vi "test TCX read (installed 71).vi"() -> ()   [LabVIEW 2011] (continued)
=\"http://www.garmin.com/xmlschemas/ActivityExtension/v2\"><Watts>106</Watts></TPX></Extensions></Trackpoint><Trackpoint><Time>2008-03-03T13:54:39Z</Time><Position><LatitudeDegrees>35.874921</LatitudeDegrees><LongitudeDegrees>-78.935340</LongitudeDegrees></Position><AltitudeMeters>93.385</AltitudeMeters><DistanceMeters>3447.353</DistanceMeters><Cadence>78</Cadence><Extensions><TPX xmlns=\"http://www.garmin.com/xmlschemas/ActivityExtension/v2\"><Watts>106</Watts></TPX></Extensions></Trackpoint><Trackpoint><Time>2008-03-03T13:54:40Z</Time><Position><LatitudeDegrees>35.874939</LatitudeDegrees><LongitudeDegrees>-78.935257</LongitudeDegrees></Position><AltitudeMeters>92.905</AltitudeMeters><DistanceMeters>3455.075</DistanceMeters><Cadence>78</Cadence><Extensions><TPX xmlns=\"http://www.garmin.com/xmlschemas/ActivityExtension/v2\"><Watts>107</Watts></TPX></Extensions></Trackpoint><Trackpoint><Time>2008-03-03T13:54:41Z</Time><Position><LatitudeDegrees>35.874959</LatitudeDegrees><LongitudeDegrees>-78.935174</LongitudeDegrees></Position><AltitudeMeters>92.905</AltitudeMeters><DistanceMeters>3462.864</DistanceMeters><Cadence>78</Cadence><Extensions><TPX xmlns=\"http://www.garmin.com/xmlschemas/ActivityExtension/v2\"><Watts>107</Watts></TPX></Extensions></Trackpoint><Trackpoint><Time>2008-03-03T13:54:42Z</Time><Position><LatitudeDegrees>35.874979</LatitudeDegrees><LongitudeDegrees>-78.935091</LongitudeDegrees></Position><AltitudeMeters>92.905</AltitudeMeters><DistanceMeters>3470.684</DistanceMeters><Cadence>79</Cadence><Extensions><TPX xmlns=\"http://www.garmin.com/xmlschemas/ActivityExtension/v2\"><Watts>102</Watts></TPX></Extensions></Trackpoint><Trackpoint><Time>2008-03-03T13:54:43Z</Time><Position><LatitudeDegrees>35.874999</LatitudeDegrees><LongitudeDegrees>-78.935010</LongitudeDegrees></Position><AltitudeMeters>92.905</AltitudeMeters><DistanceMeters>3478.419</DistanceMeters><Cadence>79</Cadence><Extensions><TPX xmlns=\"http://www.garmin.com/xmlschemas/ActivityExtension/v2\"><Watts>108</Watts></TPX></Extensions></Trackpoint><Trackpoint><Time>2008-03-03T13:54:44Z</Time><Position><LatitudeDegrees>35.875018</LatitudeDegrees><LongitudeDegrees>-78.934925</LongitudeDegrees></Position><AltitudeMeters>92.905</AltitudeMeters><DistanceMeters>3486.287</DistanceMeters><Cadence>75</Cadence><Extensions><TPX xmlns=\"http://www.garmin.com/xmlschemas/ActivityExtension/v2\"><Watts>106</Watts></TPX></Extensions></Trackpoint><Trackpoint><Time>2008-03-03T13:54:45Z</Time><Position><LatitudeDegrees>35.875035</LatitudeDegrees><LongitudeDegrees>-78.934840</LongitudeDegrees></Position><AltitudeMeters>92.424</AltitudeMeters><DistanceMeters>3494.270</DistanceMeters><Cadence>73</Cadence><Extensions><TPX xmlns=\"http://www.garmin.com/xmlschemas/ActivityExtension/v2\"><Watts>107</Watts></TPX></Extensions></Trackpoint><Trackpoint><Time>2008-03-03T13:54:46Z</Time><Position><LatitudeDegrees>35.875052</LatitudeDegrees><LongitudeDegrees>-78.934753</LongitudeDegrees></Position><AltitudeMeters>92.424</AltitudeMeters><DistanceMeters>3502.316</DistanceMeters><Cadence>73</Cadence><Extensions><TPX xmlns=\"http://www.garmin.com/xmlschemas/ActivityExtension/v2\"><Watts>109</Watts></TPX></Extensions></Trackpoint><Trackpoint><Time>2008-03-03T13:54:47Z</Time><Position><LatitudeDegrees>35.875069</LatitudeDegrees><LongitudeDegrees>-78.934665</LongitudeDegrees></Position><AltitudeMeters>92.424</AltitudeMeters><DistanceMeters>3510.458</DistanceMeters><Cadence>75</Cadence><Extensions><TPX xmlns=\"http://www.garmin.com/xmlschemas/ActivityExtension/v2\"><Watts>110</Watts></TPX></Extensions></Trackpoint><Trackpoint><Time>2008-03-03T13:54:48Z</Time><Position><LatitudeDegrees>35.875087</LatitudeDegrees><LongitudeDegrees>-78.934578</LongitudeDegrees></Position><AltitudeMeters>92.424</AltitudeMeters><DistanceMeters>3518.670</DistanceMeters><Cadence>76</Cadence><Extensions><TPX xmlns=\"http://www.garmin.com/xmlschemas/ActivityExtension/v2\"><Watts>111</Watts></TPX></Extensions></Trackpoint><Trackpoint><Time>2008-03-03T13:54:49Z</Time><Position><LatitudeDegrees>35.875104</LatitudeDegrees><LongitudeDegrees>-78.934486</LongitudeDegrees></Position><AltitudeMeters>92.424</AltitudeMeters><DistanceMeters>3527.182</DistanceMeters><Cadence>77</Cadence><Extensions><TPX xmlns=\"http://www.garmin.com/xmlschemas/ActivityExtension/v2\"><Watts>111</Watts></TPX></Extensions></Trackpoint><Trackpoint><Time>2008-03-03T13:54:50Z</Time><Position><LatitudeDegrees>35.875121</LatitudeDegrees><LongitudeDegrees>-78.934392</LongitudeDegrees></Position><AltitudeMeters>92.424</AltitudeMeters><DistanceMeters>3535.860</DistanceMeters><Cadence>79</Cadence><Extensions><TPX xmlns=\"http://www.garmin.com/xmlschemas/ActivityExtension/v2\"><Watts>111</Watts></TPX></Extensions></Trackpoint><Trackpoint><Time>2008-03-03T13:54:51Z</Time><Position><LatitudeDegrees>35.875137</LatitudeDegrees><LongitudeDegrees>-78.934295</LongitudeDegrees></Position><AltitudeMeters>91.943</AltitudeMeters><DistanceMeters>3544.788</DistanceMeters><Cadence>78</Cadence><Extensions><TPX xmlns=\"http://www.garmin.com/xmlschemas/ActivityExtension/v2\"><Watts>108</Watts></TPX></Extensions></Trackpoint><Trackpoint><Time>2008-03-03T13:54:52Z</Time><Position><LatitudeDegrees>35.875154</LatitudeDegrees><LongitudeDegrees>-78.934196</LongitudeDegrees></Position><AltitudeMeters>91.463</AltitudeMeters><DistanceMeters>3553.912</DistanceMeters><Cadence>74</Cadence><Extensions><TPX xmlns=\"http://www.garmin.com/xmlschemas/ActivityExtension/v2\"><Watts>103</Watts></TPX></Extensions></Trackpoint><Trackpoint><Time>2008-03-03T13:54:53Z</Time><Position><LatitudeDegrees>35.875172</LatitudeDegrees><LongitudeDegrees>-78.934096</LongitudeDegrees></Position><AltitudeMeters>91.463</AltitudeMeters><DistanceMeters>3563.297</DistanceMeters><Cadence>74</Cadence><Extensions><TPX xmlns=\"http://www.garmin.com/xmlschemas/ActivityExtension/v2\"><Watts>104</Watts></TPX></Extensions></Trackpoint><Trackpoint><Time>2008-03-03T13:54:54Z</Time><Position><LatitudeDegrees>35.875191</LatitudeDegrees><LongitudeDegrees>-78.933992</LongitudeDegrees></Position><AltitudeMeters>91.463</AltitudeMeters><DistanceMeters>3572.866</DistanceMeters><Cadence>77</Cadence><Extensions><TPX xmlns=\"http://www.garmin.com/xmlschemas/ActivityExtension/v2\"><Watts>118</Watts></TPX></Extensions></Trackpoint><Trackpoint><Time>2008-03-03T13:54:55Z</Time><Position><LatitudeDegrees>35.875211</LatitudeDegrees><LongitudeDegrees>-78.933885</LongitudeDegrees></Position><AltitudeMeters>90.982</AltitudeMeters><DistanceMeters>3582.741</DistanceMeters><Cadence>77</Cadence><Extensions><TPX xmlns=\"http://www.garmin.com/xmlschemas/ActivityExtension/v2\"><Watts>116</Watts></TPX></Extensions></Trackpoint><Trackpoint><Time>2008-03-03T13:54:56Z</Time><Position><LatitudeDegrees>35.875231</LatitudeDegrees><LongitudeDegrees>-78.933776</LongitudeDegrees></Position><AltitudeMeters>90.501</AltitudeMeters><DistanceMeters>3592.905</DistanceMeters><Cadence>73</Cadence><Extensions><TPX xmlns=\"http://www.garmin.com/xmlschemas/ActivityExtension/v2\"><Watts>109</Watts></TPX></Extensions></Trackpoint><Trackpoint><Time>2008-03-03T13:54:57Z</Time><Position><LatitudeDegrees>35.875253</LatitudeDegrees><LongitudeDegrees>-78.933665</LongitudeDegrees></Position><AltitudeMeters>90.501</AltitudeMeters><DistanceMeters>3603.271</DistanceMeters><Cadence>74</Cadence><Extensions><TPX xmlns=\"http://www.garmin.com/xmlschemas/ActivityExtension/v2\"><Watts>116</Watts></TPX></Extensions></Trackpoint><Trackpoint><Time>2008-03-03T13:54:58Z</Time><Position><LatitudeDegrees>35.875274</LatitudeDegrees><LongitudeDegrees>-78.933548</LongitudeDegrees></Position><AltitudeMeters>89.540</AltitudeMeters><DistanceMeters>3614.042</DistanceMeters><Cadence>74</Cadence><Extensions><TPX xmlns=\"http://www.garmin.com/xmlschemas/ActivityExtension/v2\"><Watts>115</Watts></TPX></Extensions></Trackpoint><Trackpoint><Time>2008-03-03T13:54:59Z</Time><Position><LatitudeDegrees>35.875302</LatitudeDegrees><LongitudeDegrees>-78.933428</LongitudeDegrees></Position><AltitudeMeters>88.579</AltitudeMeters><DistanceMeters>3625.394</DistanceMeters><Cadence>77</Cadence><Extensions><TPX xmlns=\"http://www.garmin.com/xmlschemas/ActivityExtension/v2\"><Watts>111</Watts></TPX></Extensions></Trackpoint><Trackpoint><Time>2008-03-03T13:55:00Z</Time><Position><LatitudeDegrees>35.875328</LatitudeDegrees><LongitudeDegrees>-78.933302</LongitudeDegrees></Position><AltitudeMeters>87.617</AltitudeMeters><DistanceMeters>3637.135</DistanceMeters><Cadence>83</Cadence><Extensions><TPX xmlns=\"http://www.garmin.com/xmlschemas/ActivityExtension/v2\"><Watts>111</Watts></TPX></Extensions></Trackpoint><Trackpoint><Time>2008-03-03T13:55:01Z</Time><Position><LatitudeDegrees>35.875352</LatitudeDegrees><LongitudeDegrees>-78.933170</LongitudeDegrees></Position><AltitudeMeters>86.656</AltitudeMeters><DistanceMeters>3649.341</DistanceMeters><Cadence>87</Cadence><Extensions><TPX xmlns=\"http://www.garmin.com/xmlschemas/ActivityExtension/v2\"><Watts>108</Watts></TPX></Extensions></Trackpoint><Trackpoint><Time>2008-03-03T13:55:02Z</Time><Position><LatitudeDegrees>35.875375</LatitudeDegrees><LongitudeDegrees>-78.933034</LongitudeDegrees></Position><AltitudeMeters>86.175</AltitudeMeters><DistanceMeters>3661.935</DistanceMeters><Cadence>77</Cadence><Extensions><TPX xmlns=\"http://www.garmin.com/xmlschemas/ActivityExtension/v2\"><Watts>105</Watts></TPX></Extensions></Trackpoint><Trackpoint><Time>2008-03-03T13:55:03Z</Time><Position><LatitudeDegrees>35.875397</LatitudeDegrees><LongitudeDegrees>-78.932892</LongitudeDegrees></Position><AltitudeMeters>85.695</AltitudeMeters><DistanceMeters>3675.075</DistanceMeters><Cadence>77</Cadence><Extensions><TPX xmlns=\"http://www.garmin.com/xmlschemas/ActivityExtension/v2\"><Watts>106</Watts></TPX></Extensions></Trackpoint><Trackpoint><Time>2008-03-03T13:55:04Z</Time><Position><LatitudeDegrees>35.875423</LatitudeDegrees><LongitudeDegrees>-78.932744</LongitudeDegrees></Position><AltitudeMeters>84.733</AltitudeMeters><DistanceMeters>3688.721</DistanceMeters><Cadence>81</Cadence><Extensions><TPX xmlns=\"http://www.garmin.com/xmlschemas/ActivityExtension/v2\"><Watts>109</Watts></TPX></Extensions></Trackpoint><Trackpoint><Time>2008-03-03T13:55:05Z</Time><Position><LatitudeDegrees>35.875451</LatitudeDegrees><LongitudeDegrees>-78.932591</LongitudeDegrees></Position><AltitudeMeters>83.772</AltitudeMeters><DistanceMeters>3702.913</DistanceMeters><Cadence>84</Cadence><Extensions><TPX xmlns=\"http://www.garmin.com/xmlschemas/ActivityExtension/v2\"><Watts>130</Watts></TPX></Extensions></Trackpoint><Trackpoint><Time>2008-03-03T13:55:06Z</Time><Position><LatitudeDegrees>35.875484</LatitudeDegrees><LongitudeDegrees>-78.932435</LongitudeDegrees></Position><AltitudeMeters>83.291</AltitudeMeters><DistanceMeters>3717.524</DistanceMeters><Cadence>87</Cadence><Extensions><TPX xmlns=\"http://www.garmin.com/xmlschemas/ActivityExtension/v2\"><Watts>156</Watts></TPX></Extensions></Trackpoint><Trackpoint><Time>2008-03-03T13:55:07Z</Time><Position><LatitudeDegrees>35.875516</LatitudeDegrees><LongitudeDegrees>-78.932275</LongitudeDegrees></Position><AltitudeMeters>82.811</AltitudeMeters><DistanceMeters>3732.393</DistanceMeters><Cadence>89</Cadence><Extensions><TPX xmlns=\"http://www.garmin.com/xmlschemas/ActivityExtension/v2\"><Watts>168</Watts></TPX></Extensions></Trackpoint><Trackpoint><Time>2008-03-03T13:55:08Z</Time><Position><LatitudeDegrees>35.875546</LatitudeDegrees><LongitudeDegrees>-78.932113</LongitudeDegrees></Position><AltitudeMeters>81.849</AltitudeMeters><DistanceMeters>3747.414</DistanceMeters><Cadence>90</Cadence><Extensions><TPX xmlns=\"http://www.garmin.com/xmlschemas/ActivityExtension/v2\"><Watts>157</Watts></TPX></Extensions></Trackpoint><Trackpoint><Time>2008-03-03T13:55:09Z</Time><Position><LatitudeDegrees>35.875574</LatitudeDegrees><LongitudeDegrees>-78.931949</LongitudeDegrees></Position><AltitudeMeters>80.888</AltitudeMeters><DistanceMeters>3762.486</DistanceMeters><Cadence>89</Cadence><Extensions><TPX xmlns=\"http://www.garmin.com/xmlschemas/ActivityExtension/v2\"><Watts>146</Watts></TPX></Extensions></Trackpoint><Trackpoint><Time>2008-03-03T13:55:10Z</Time><Position><LatitudeDegrees>35.875600</LatitudeDegrees><LongitudeDegrees>-78.931785</LongitudeDegrees></Position><AltitudeMeters>80.407</AltitudeMeters><DistanceMeters>3777.574</DistanceMeters><Cadence>89</Cadence><Extensions><TPX xmlns=\"http://www.garmin.com/xmlschemas/ActivityExtension/v2\"><Watts>134</Watts></TPX></Extensions></Trackpoint><Trackpoint><Time>2008-03-03T13:55:11Z</Time><Position><LatitudeDegrees>35.875627</LatitudeDegrees><LongitudeDegrees>-78.931623</LongitudeDegrees></Position><AltitudeMeters>79.446</AltitudeMeters><DistanceMeters>3792.520</DistanceMeters><Cadence>89</Cadence><Extensions><TPX xmlns=\"http://www.garmin.com/xmlschemas/ActivityExtension/v2\"><Watts>130</Watts></TPX></Extensions></Trackpoint><Trackpoint><Time>2008-03-03T13:55:12Z</Time><Position><LatitudeDegrees>35.875652</LatitudeDegrees><LongitudeDegrees>-78.931459</LongitudeDegrees></Position><AltitudeMeters>79.446</AltitudeMeters><DistanceMeters>3807.590</DistanceMeters><Cadence>88</Cadence><Extensions><TPX xmlns=\"http://www.garmin.com/xmlschemas/ActivityExtension/v2\"><Watts>124</Watts></TPX></Extensions></Trackpoint><Trackpoint><Time>2008-03-03T13:55:13Z</Time><Position><LatitudeDegrees>35.875671</LatitudeDegrees><LongitudeDegrees>-78.931297</LongitudeDegrees></Position><AltitudeMeters>78.965</AltitudeMeters><DistanceMeters>3822.386</DistanceMeters><Cadence>88</Cadence><Extensions><TPX xmlns=\"http://www.garmin.com/xmlschemas/ActivityExtension/v2\"><Watts>124</Watts></TPX></Extensions></Trackpoint><Trackpoint><Time>2008-03-03T13:55:14Z</Time><Position><LatitudeDegrees>35.875682</LatitudeDegrees><LongitudeDegrees>-78.931138</LongitudeDegrees></Position><AltitudeMeters>78.004</AltitudeMeters><DistanceMeters>3836.777</DistanceMeters><Cadence>86</Cadence><Extensions><TPX xmlns=\"http://www.garmin.com/xmlschemas/ActivityExtension/v2\"><Watts>122</Watts></TPX></Extensions></Trackpoint><Trackpoint><Time>2008-03-03T13:55:15Z</Time><Position><LatitudeDegrees>35.875686</LatitudeDegrees><LongitudeDegrees>-78.930981</LongitudeDegrees></Position><AltitudeMeters>78.004</AltitudeMeters><DistanceMeters>3850.902</DistanceMeters><Cadence>85</Cadence><Extensions><TPX xmlns=\"http://www.garmin.com/xmlschemas/ActivityExtension/v2\"><Watts>136</Watts></TPX></Extensions></Trackpoint><Trackpoint><Time>2008-03-03T13:55:16Z</Time><Position><LatitudeDegrees>35.875685</LatitudeDegrees><LongitudeDegrees>-78.930828</LongitudeDegrees></Position><AltitudeMeters>78.004</AltitudeMeters><DistanceMeters>3864.689</DistanceMeters><Cadence>83</Cadence><Extensions><TPX xmlns=\"http://www.garmin.com/xmlschemas/ActivityExtension/v2\"><Watts>148</Watts></TPX></Extensions></Trackpoint><Trackpoint><Time>2008-03-03T13:55:17Z</Time><Position><LatitudeDegrees>35.875684</LatitudeDegrees><LongitudeDegrees>-78.930679</LongitudeDegrees></Position><AltitudeMeters>77.523</AltitudeMeters><DistanceMeters>3878.168</DistanceMeters><Cadence>80</Cadence><Extensions><TPX xmlns=\"http://www.garmin.com/xmlschemas/ActivityExtension/v2\"><Watts>165</Watts></TPX></Extensions></Trackpoint><Trackpoint><Time>2008-03-03T13:55:18Z</Time><Position><LatitudeDegrees>35.875681</LatitudeDegrees><LongitudeDegrees>-78.930532</LongitudeDegrees></Position><AltitudeMeters>77.043</AltitudeMeters><DistanceMeters>3891.426</DistanceMeters><Cadence>79</Cadence><Extensions><TPX xmlns=\"http://www.garmin.com/xmlschemas/ActivityExtension/v2\"><Watts>164</Watts></TPX></Extensions></Trackpoint><Trackpoint><Time>2008-03-03T13:55:19Z</Time><Position><LatitudeDegrees>35.875675</LatitudeDegrees><LongitudeDegrees>-78.930389</LongitudeDegrees></Position><AltitudeMeters>77.043</AltitudeMeters><DistanceMeters>3904.342</DistanceMeters><Cadence>78</Cadence><Extensions><TPX xmlns=\"http://www.garmin.com/xmlschemas/ActivityExtension/v2\"><Watts>161</Watts></TPX></Extensions></Trackpoint><Trackpoint><Time>2008-03-03T13:55:20Z</Time><Position><LatitudeDegrees>35.875671</LatitudeDegrees><LongitudeDegrees>-78.930247</LongitudeDegrees></Position><AltitudeMeters>76.562</AltitudeMeters><DistanceMeters>3917.112</DistanceMeters><Cadence>76</Cadence><Extensions><TPX xmlns=\"http://www.garmin.com/xmlschemas/ActivityExtension/v2\"><Watts>154</Watts></TPX></Extensions></Trackpoint><Trackpoint><Time>2008-03-03T13:55:21Z</Time><Position><LatitudeDegrees>35.875667</LatitudeDegrees><LongitudeDegrees>-78.930109</LongitudeDegrees></Position><AltitudeMeters>78.004</AltitudeMeters><DistanceMeters>3929.621</DistanceMeters><Cadence>75</Cadence><Extensions><TPX xmlns=\"http://www.garmin.com/xmlschemas/ActivityExtension/v2\"><Watts>160</Watts></TPX></Extensions></Trackpoint><Trackpoint><Time>2008-03-03T13:55:22Z</Time><Position><LatitudeDegrees>35.875662</LatitudeDegrees><LongitudeDegrees>-78.929972</LongitudeDegrees></Position><AltitudeMeters>77.043</AltitudeMeters><DistanceMeters>3941.995</DistanceMeters><Cadence>74</Cadence><Extensions><TPX xmlns=\"http://www.garmin.com/xmlschemas/ActivityExtension/v2\"><Watts>164</Watts></TPX></Extensions></Trackpoint><Trackpoint><Time>2008-03-03T13:55:23Z</Time><Position><LatitudeDegrees>35.875657</LatitudeDegrees><LongitudeDegrees>-78.929836</LongitudeDegrees></Position><AltitudeMeters>76.562</AltitudeMeters><DistanceMeters>3954.253</DistanceMeters><Cadence>74</Cadence><Extensions><TPX xmlns=\"http://www.garmin.com/xmlschemas/ActivityExtension/v2\"><Watts>162</Watts></TPX></Extensions></Trackpoint><Trackpoint><Time>2008-03-03T13:55:24Z</Time><Position><LatitudeDegrees>35.875652</LatitudeDegrees><LongitudeDegrees>-78.929703</LongitudeDegrees></Position><AltitudeMeters>76.562</AltitudeMeters><DistanceMeters>3966.223</DistanceMeters><Cadence>72</Cadence><Extensions><TPX xmlns=\"http://www.garmin.com/xmlschemas/ActivityExtension/v2\"><Watts>178</Watts></TPX></Extensions></Trackpoint><Trackpoint><Time>2008-03-03T13:55:25Z</Time><Position><LatitudeDegrees>35.875651</LatitudeDegrees><LongitudeDegrees>-78.929573</LongitudeDegrees></Position><AltitudeMeters>76.081</AltitudeMeters><DistanceMeters>3978.047</DistanceMeters><Cadence>72</Cadence><Extensions><TPX xmlns=\"http://www.garmin.com/xmlschemas/ActivityExtension/v2\"><Watts>180</Watts></TPX></Extensions></Trackpoint><Trackpoint><Time>2008-03-03T13:55:26Z</Time><Position><LatitudeDegrees>35.875647</LatitudeDegrees><LongitudeDegrees>-78.929443</LongitudeDegrees></Position><AltitudeMeters>76.081</AltitudeMeters><DistanceMeters>3989.714</DistanceMeters><Cadence>71</Cadence><Extensions><TPX xmlns=\"http://www.garmin.com/xmlschemas/ActivityExtension/v2\"><Watts>192</Watts></TPX></Extensions></Trackpoint><Trackpoint><Time>2008-03-03T13:55:27Z</Time><Position><LatitudeDegrees>35.875640</LatitudeDegrees><LongitudeDegrees>-78.929316</LongitudeDegrees></Position><AltitudeMeters>76.562</AltitudeMeters><DistanceMeters>4001.237</DistanceMeters><Cadence>69</Cadence><Extensions><TPX xmlns=\"http://www.garmin.com/xmlschemas/ActivityExtension/v2\"><Watts>191</Watts></TPX></Extensions></Trackpoint><Trackpoint><Time>2008-03-03T13:55:28Z</Time><Position><LatitudeDegrees>35.875631</LatitudeDegrees><LongitudeDegrees>-78.929192</LongitudeDegrees></Position><AltitudeMeters>77.043</AltitudeMeters><DistanceMeters>4012.524</DistanceMeters><Cadence>68</Cadence><Extensions><TPX xmlns=\"http://www.garmin.com/xmlschemas/ActivityExtension/v2\"><Watts>166</Watts></TPX></Extensions></Trackpoint><Trackpoint><Time>2008-03-03T13:55:29Z</Time><Position><LatitudeDegrees>35.875625</LatitudeDegrees><LongitudeDegrees>-78.929072</LongitudeDegrees></Position><AltitudeMeters>77.043</AltitudeMeters><DistanceMeters>4023.291</DistanceMeters><Cadence>66</Cadence><Extensions><TPX xmlns=\"http://www.garmin.com/xmlschemas/ActivityExtension/v2\"><Watts>142</Watts></TPX></Extensions></Trackpoint><Trackpoint><Time>2008-03-03T13:55:30Z</Time><Position><LatitudeDegrees>35.875618</LatitudeDegrees><LongitudeDegrees>-78.928955</LongitudeDegrees></Position><AltitudeMeters>76.562</AltitudeMeters><DistanceMeters>4033.810</DistanceMeters><Cadence>66</Cadence><Extensions><TPX xmlns=\"http://www.garmin.com/xmlschemas/ActivityExtension/v2\"><Watts>142</Watts></TPX></Extensions></Trackpoint><Trackpoint><Time>2008-03-03T13:55:31Z</Time><Position><LatitudeDegrees>35.875612</LatitudeDegrees><LongitudeDegrees>-78.928844</LongitudeDegrees></Position><AltitudeMeters>76.562</AltitudeMeters><DistanceMeters>4043.911</DistanceMeters><Cadence>68</Cadence><Extensions><TPX xmlns=\"http://www.garmin.com/xmlschemas/ActivityExtension/v2\"><Watts>145</Watts></TPX></Extensions></Trackpoint><Trackpoint><Time>2008-03-03T13:55:32Z</Time><Position><LatitudeDegrees>35.875608</LatitudeDegrees><LongitudeDegrees>-78.928738</LongitudeDegrees></Position><AltitudeMeters>77.043</AltitudeMeters><DistanceMeters>4053.442</DistanceMeters><Cadence>68</Cadence><Extensions><TPX xmlns=\"http://www.garmin.com/xmlschemas/ActivityExtension/v2\"><Watts>151</Watts></TPX></Extensions></Trackpoint><Trackpoint><Time>2008-03-03T13:55:33Z</Time><Position><LatitudeDegrees>35.875606</LatitudeDegrees><LongitudeDegrees>-78.928635</LongitudeDegrees></Position><AltitudeMeters>77.523</AltitudeMeters><DistanceMeters>4062.742</DistanceMeters><Cadence>68</Cadence><Extensions><TPX xmlns=\"http://www.garmin.com/xmlschemas/ActivityExtension/v2\"><Watts>149</Watts></TPX></Extensions></Trackpoint><Trackpoint><Time>2008-03-03T13:55:34Z</Time><Position><LatitudeDegrees>35.875603</LatitudeDegrees><LongitudeDegrees>-78.928536</LongitudeDegrees></Position><AltitudeMeters>78.004</AltitudeMeters><DistanceMeters>4071.697</DistanceMeters><Cadence>65</Cadence><Extensions><TPX xmlns=\"http://www.garmin.com/xmlschemas/ActivityExtension/v2\"><Watts>312</Watts></TPX></Extensions></Trackpoint><Trackpoint><Time>2008-03-03T13:55:35Z</Time><Position><LatitudeDegrees>35.875600</LatitudeDegrees><LongitudeDegrees>-78.928438</LongitudeDegrees></Position><AltitudeMeters>78.485</AltitudeMeters><DistanceMeters>4080.494</DistanceMeters><Cadence>65</Cadence><Extensions><TPX xmlns=\"http://www.garmin.com/xmlschemas/ActivityExtension/v2\"><Watts>316</Watts></TPX></Extensions></Trackpoint><Trackpoint><Time>2008-03-03T13:55:36Z</Time><Position><LatitudeDegrees>35.875592</LatitudeDegrees><LongitudeDegrees>-78.928342</LongitudeDegrees></Position><AltitudeMeters>78.485</AltitudeMeters><DistanceMeters>4089.234</DistanceMeters><Cadence>63</Cadence><Extensions><TPX xmlns=\"http://www.garmin.com/xmlschemas/ActivityExtension/v2\"><Watts>338</Watts></TPX></Extensions></Trackpoint><Trackpoint><Time>2008-03-03T13:55:37Z</Time><Position><LatitudeDegrees>35.875583</LatitudeDegrees><LongitudeDegrees>-78.928247</LongitudeDegrees></Position><AltitudeMeters>78.965</AltitudeMeters><DistanceMeters>4097.860</DistanceMeters><Cadence>62</Cadence><Extensions><TPX xmlns=\"http://www.garmin.com/xmlschemas/ActivityExtension/v2\"><Watts>355</Watts></TPX></Extensions></Trackpoint><Trackpoint><Time>2008-03-03T13:55:38Z</Time><Position><LatitudeDegrees>35.875580</LatitudeDegrees><LongitudeDegrees>-78.928153</LongitudeDegrees></Position><AltitudeMeters>79.446</AltitudeMeters><DistanceMeters>4106.294</DistanceMeters><Cadence>61</Cadence><Extensions><TPX xmlns=\"http://www.garmin.com/xmlschemas/ActivityExtension/v2\"><Watts>372</Watts></TPX></Extensions></Trackpoint><Trackpoint><Time>2008-03-03T13:55:39Z</Time><Position><LatitudeDegrees>35.875570</LatitudeDegrees><LongitudeDegrees>-78.928059</LongitudeDegrees></Position><AltitudeMeters>79.446</AltitudeMeters><DistanceMeters>4114.865</DistanceMeters><Cadence>61</Cadence><Extensions><TPX xmlns=\"http://www.garmin.com/xmlschemas/ActivityExtension/v2\"><Watts>376</Watts></TPX></Extensions></Trackpoint><Trackpoint><Time>2008-03-03T13:55:40Z</Time><Position><LatitudeDegrees>35.875562</LatitudeDegrees><LongitudeDegrees>-78.927965</LongitudeDegrees></Position><AltitudeMeters>79.927</AltitudeMeters><DistanceMeters>4123.438</DistanceMeters><Cadence>61</Cadence><Extensions><TPX xmlns=\"http://www.garmin.com/xmlschemas/ActivityExtension/v2\"><Watts>374</Watts></TPX></Extensions></Trackpoint><Trackpoint><Time>2008-03-03T13:55:41Z</Time><Position><LatitudeDegrees>35.875555</LatitudeDegrees><LongitudeDegrees>-78.927871</LongitudeDegrees></Position><AltitudeMeters>79.927</AltitudeMeters><DistanceMeters>4131.906</DistanceMeters><Cadence>61</Cadence><Extensions><TPX xmlns=\"http://www.garmin.com/xmlschemas/ActivityExtension/v2\"><Watts>375</Watts></TPX></Extensions></Trackpoint><Trackpoint><Time>2008-03-03T13:55:42Z</Time><Position><LatitudeDegrees>35.875548</LatitudeDegrees><LongitudeDegrees>-78.927776</LongitudeDegrees></Position><AltitudeMeters>79.927</AltitudeMeters><DistanceMeters>4140.581</DistanceMeters><Cadence>62</Cadence><Extensions><TPX xmlns=\"http://www.garmin.com/xmlschemas/ActivityExtension/v2\"><Watts>335</Watts></TPX></Extensions></Trackpoint><Trackpoint><Time>2008-03-03T13:55:43Z</Time><Position><LatitudeDegrees>35.875543</LatitudeDegrees><LongitudeDegrees>-78.927681</LongitudeDegrees></Position><AltitudeMeters>80.407</AltitudeMeters><DistanceMeters>4149.183</DistanceMeters><Cadence>62</Cadence><Extensions><TPX xmlns=\"http://www.garmin.com/xmlschemas/ActivityExtension/v2\"><Watts>289</Watts></TPX></Extensions></Trackpoint><Trackpoint><Time>2008-03-03T13:55:44Z</Time><Position><LatitudeDegrees>35.875535</LatitudeDegrees><LongitudeDegrees>-78.927586</LongitudeDegrees></Position><AltitudeMeters>80.407</AltitudeMeters><DistanceMeters>4157.797</DistanceMeters><Cadence>62</Cadence><Extensions><TPX xmlns=\"http://www.garmin.com/xmlschemas/ActivityExtension/v2\"><Watts>224</Watts></TPX></Extensions></Trackpoint><Trackpoint><Time>2008-03-03T13:55:45Z</Time><Position><LatitudeDegrees>35.875521</LatitudeDegrees><LongitudeDegrees>-78.927489</LongitudeDegrees></Position><AltitudeMeters>80.407</AltitudeMeters><DistanceMeters>4166.648</DistanceMeters><Cadence>62</Cadence><Extensions><TPX xmlns=\"http://www.garmin.com/xmlschemas/ActivityExtension/v2\"><Watts>223</Watts></TPX></Extensions></Trackpoint><Trackpoint><Time>2008-03-03T13:55:46Z</Time><Position><LatitudeDegrees>35.875508</LatitudeDegrees><LongitudeDegrees>-78.927391</LongitudeDegrees></Position><AltitudeMeters>79.927</AltitudeMeters><DistanceMeters>4175.647</DistanceMeters><Cadence>63</Cadence><Extensions><TPX xmlns=\"http://www.garmin.com/xmlschemas/ActivityExtension/v2\"><Watts>210</Watts></TPX></Extensions></Trackpoint><Trackpoint><Time>2008-03-03T13:55:47Z</Time><Position><LatitudeDegrees>35.875496</LatitudeDegrees><LongitudeDegrees>-78.927292</LongitudeDegrees></Position><AltitudeMeters>79.927</AltitudeMeters><DistanceMeters>4184.702</DistanceMeters><Cadence>63</Cadence><Extensions><TPX xmlns=\"http://www.garmin.com/xmlschemas/ActivityExtension/v2\"><Watts>206</Watts></TPX></Extensions></Trackpoint><Trackpoint><Time>2008-03-03T13:55:48Z</Time><Position><LatitudeDegrees>35.875484</LatitudeDegrees><LongitudeDegrees>-78.927191</LongitudeDegrees></Position><AltitudeMeters>79.927</AltitudeMeters><DistanceMeters>4193.944</DistanceMeters><Cadence>64</Cadence><Extensions><TPX xmlns=\"http://www.garmin.com/xmlschemas/ActivityExtension/v2\"><Watts>175</Watts></TPX></Extensions></Trackpoint><Trackpoint><Time>2008-03-03T13:55:49Z</Time><Position><LatitudeDegrees>35.875472</LatitudeDegrees><LongitudeDegrees>-78.927087</LongitudeDegrees></Position><AltitudeMeters>78.965</AltitudeMeters><DistanceMeters>4203.405</DistanceMeters><Cadence>67</Cadence><Extensions><TPX xmlns=\"http://www.garmin.com/xmlschemas/ActivityExtension/v2\"><Watts>118</Watts></TPX></Extensions></Trackpoint><Trackpoint><Time>2008-03-03T13:55:50Z</Time><Position><LatitudeDegrees>35.875459</LatitudeDegrees><LongitudeDegrees>-78.926981</LongitudeDegrees></Position><AltitudeMeters>79.446</AltitudeMeters><DistanceMeters>4213.108</DistanceMeters><Cadence>69</Cadence><Extensions><TPX xmlns=\"http://www.garmin.com/xmlschemas/ActivityExtension/v2\"><Watts>109</Watts></TPX></Extensions></Trackpoint><Trackpoint><Time>2008-03-03T13:55:51Z</Time><Position><LatitudeDegrees>35.875446</LatitudeDegrees><LongitudeDegrees>-78.926870</LongitudeDegrees></Position><AltitudeMeters>78.485</AltitudeMeters><DistanceMeters>4223.207</DistanceMeters><Cadence>71</Cadence><Extensions><TPX xmlns=\"http://www.garmin.com/xmlschemas/ActivityExtension/v2\"><Watts>106</Watts></TPX></Extensions></Trackpoint><Trackpoint><Time>2008-03-03T13:55:52Z</Time><Position><LatitudeDegrees>35.875433</LatitudeDegrees><LongitudeDegrees>-78.926755</LongitudeDegrees></Position><AltitudeMeters>78.485</AltitudeMeters><DistanceMeters>4233.738</DistanceMeters><Cadence>71</Cadence><Extensions><TPX xmlns=\"http://www.garmin.com/xmlschemas/ActivityExtension/v2\"><Watts>107</Watts></TPX></Extensions></Trackpoint><Trackpoint><Time>2008-03-03T13:55:53Z</Time><Position><LatitudeDegrees>35.875420</LatitudeDegrees><LongitudeDegrees>-78.926635</LongitudeDegrees></Position><AltitudeMeters>78.004</AltitudeMeters><DistanceMeters>4244.720</DistanceMeters><Cadence>79</Cadence><Extensions><TPX xmlns=\"http://www.garmin.com/xmlschemas/ActivityExtension/v2\"><Watts>106</Watts></TPX></Extensions></Trackpoint><Trackpoint><Time>2008-03-03T13:55:54Z</Time><Position><LatitudeDegrees>35.875406</LatitudeDegrees><LongitudeDegrees>-78.926511</LongitudeDegrees></Position><AltitudeMeters>77.043</AltitudeMeters><DistanceMeters>4256.063</DistanceMeters><Cadence>81</Cadence><Extensions><TPX xmlns=\"http://www.garmin.com/xmlschemas/ActivityExtension/v2\"><Watts>108</Watts></TPX></Extensions></Trackpoint><Trackpoint><Time>2008-03-03T13:55:55Z</Time><Position><LatitudeDegrees>35.875394</LatitudeDegrees><LongitudeDegrees>-78.926382</LongitudeDegrees></Position><AltitudeMeters>76.562</AltitudeMeters><DistanceMeters>4267.799</DistanceMeters><Cadence>84</Cadence><Extensions><TPX xmlns=\"http://www.garmin.com/xmlschemas/ActivityExtension/v2\"><Watts>102</Watts></TPX></Extensions></Trackpoint><Trackpoint><Time>2008-03-03T13:55:56Z</Time><Position><LatitudeDegrees>35.875387</LatitudeDegrees><LongitudeDegrees>-78.926251</LongitudeDegrees></Position><AltitudeMeters>76.562</AltitudeMeters><DistanceMeters>4279.712</DistanceMeters><Cadence>85</Cadence><Extensions><TPX xmlns=\"http://www.garmin.com/xmlschemas/ActivityExtension/v2\"><Watts>103</Watts></TPX></Extensions></Trackpoint><Trackpoint><Time>2008-03-03T13:55:57Z</Time><Position><LatitudeDegrees>35.875381</LatitudeDegrees><LongitudeDegrees>-78.926117</LongitudeDegrees></Position><AltitudeMeters>76.562</AltitudeMeters><DistanceMeters>4291.779</DistanceMeters><Cadence>85</Cadence><Extensions><TPX xmlns=\"http://www.garmin.com/xmlschemas/ActivityExtension/v2\"><Watts>102</Watts></TPX></Extensions></Trackpoint><Trackpoint><Time>2008-03-03T13:55:58Z</Time><Position><LatitudeDegrees>35.875374</LatitudeDegrees><LongitudeDegrees>-78.925982</LongitudeDegrees></Position><AltitudeMeters>76.081</AltitudeMeters><DistanceMeters>4304.011</DistanceMeters><Cadence>85</Cadence><Extensions><TPX xmlns=\"http://www.garmin.com/xmlschemas/ActivityExtension/v2\"><Watts>107</Watts></TPX></Extensions></Trackpoint><Trackpoint><Time>2008-03-03T13:55:59Z</Time><Position><LatitudeDegrees>35.875372</LatitudeDegrees><LongitudeDegrees>-78.925849</LongitudeDegrees></Position><AltitudeMeters>75.120</AltitudeMeters><DistanceMeters>4316.005</DistanceMeters><Cadence>84</Cadence><Extensions><TPX xmlns=\"http://www.garmin.com/xmlschemas/ActivityExtension/v2\"><Watts>105</Watts></TPX></Extensions></Trackpoint><Trackpoint><Time>2008-03-03T13:56:00Z</Time><Position><LatitudeDegrees>35.875374</LatitudeDegrees><LongitudeDegrees>-78.925719</LongitudeDegrees></Position><AltitudeMeters>74.640</AltitudeMeters><DistanceMeters>4327.800</DistanceMeters><Cadence>83</Cadence><Extensions><TPX xmlns=\"http://www.garmin.com/xmlschemas/ActivityExtension/v2\"><Watts>108</Watts></TPX></Extensions></Trackpoint><Trackpoint><Time>2008-03-03T13:56:01Z</Time><Position><LatitudeDegrees>35.875377</LatitudeDegrees><LongitudeDegrees>-78.925590</LongitudeDegrees></Position><AltitudeMeters>74.640</AltitudeMeters><DistanceMeters>4339.303</DistanceMeters><Cadence>81</Cadence><Extensions><TPX xmlns=\"http://www.garmin.com/xmlschemas/ActivityExtension/v2\"><Watts>111</Watts></TPX></Extensions></Trackpoint><Trackpoint><Time>2008-03-03T13:56:02Z</Time><Position><LatitudeDegrees>35.875376</LatitudeDegrees><LongitudeDegrees>-78.925464</LongitudeDegrees></Position><AltitudeMeters>74.159</AltitudeMeters><DistanceMeters>4350.667</DistanceMeters><Cadence>81</Cadence><Extensions><TPX xmlns=\"http://www.garmin.com/xmlschemas/ActivityExtension/v2\"><Watts>110</Watts></TPX></Extensions></Trackpoint><Trackpoint><Time>2008-03-03T13:56:03Z</Time><Position><LatitudeDegrees>35.875378</LatitudeDegrees><LongitudeDegrees>-78.925342</LongitudeDegrees></Position><AltitudeMeters>74.640</AltitudeMeters><DistanceMeters>4361.797</DistanceMeters><Cadence>79</Cadence><Extensions><TPX xmlns=\"http://www.garmin.com/xmlschemas/ActivityExtension/v2\"><Watts>111</Watts></TPX></Extensions></Trackpoint><Trackpoint><Time>2008-03-03T13:56:04Z</Time><Position><LatitudeDegrees>35.875384</LatitudeDegrees><LongitudeDegrees>-78.925223</LongitudeDegrees></Position><AltitudeMeters>74.640</AltitudeMeters><DistanceMeters>4372.489</DistanceMeters><Cadence>76</Cadence><Extensions><TPX xmlns=\"http://www.garmin.com/xmlschemas/ActivityExtension/v2\"><Watts>110</Watts></TPX></Extensions></Trackpoint><Trackpoint><Time>2008-03-03T13:56:05Z</Time><Position><LatitudeDegrees>35.875386</LatitudeDegrees><LongitudeDegrees>-78.925107</LongitudeDegrees></Position><AltitudeMeters>74.640</AltitudeMeters><DistanceMeters>4382.901</DistanceMeters><Cadence>73</Cadence><Extensions><TPX xmlns=\"http://www.garmin.com/xmlschemas/ActivityExtension/v2\"><Watts>108</Watts></TPX></Extensions></Trackpoint><Trackpoint><Time>2008-03-03T13:56:06Z</Time><Position><LatitudeDegrees>35.875385</LatitudeDegrees><LongitudeDegrees>-78.924996</LongitudeDegrees></Position><AltitudeMeters>74.640</AltitudeMeters><DistanceMeters>4392.956</DistanceMeters><Cadence>70</Cadence><Extensions><TPX xmlns=\"http://www.garmin.com/xmlschemas/ActivityExtension/v2\"><Watts>107</Watts></TPX></Extensions></Trackpoint><Trackpoint><Time>2008-03-03T13:56:07Z</Time><Position><LatitudeDegrees>35.875383</LatitudeDegrees><LongitudeDegrees>-78.924890</LongitudeDegrees></Position><AltitudeMeters>75.120</AltitudeMeters><DistanceMeters>4402.532</DistanceMeters><Cadence>68</Cadence><Extensions><TPX xmlns=\"http://www.garmin.com/xmlschemas/ActivityExtension/v2\"><Watts>121</Watts></TPX></Extensions></Trackpoint><Trackpoint><Time>2008-03-03T13:56:08Z</Time><Position><LatitudeDegrees>35.875378</LatitudeDegrees><LongitudeDegrees>-78.924787</LongitudeDegrees></Position><AltitudeMeters>75.120</AltitudeMeters><DistanceMeters>4411.806</DistanceMeters><Cadence>65</Cadence><Extensions><TPX xmlns=\"http://www.garmin.com/xmlschemas/ActivityExtension/v2\"><Watts>135</Watts></TPX></Extensions></Trackpoint><Trackpoint><Time>2008-03-03T13:56:09Z</Time><Position><LatitudeDegrees>35.875376</LatitudeDegrees><LongitudeDegrees>-78.924688</LongitudeDegrees></Position><AltitudeMeters>75.601</AltitudeMeters><DistanceMeters>4420.687</DistanceMeters><Cadence>67</Cadence><Extensions><TPX xmlns=\"http://www.garmin.com/xmlschemas/ActivityExtension/v2\"><Watts>138</Watts></TPX></Extensions></Trackpoint><Trackpoint><Time>2008-03-03T13:56:10Z</Time><Position><LatitudeDegrees>35.875376</LatitudeDegrees><LongitudeDegrees>-78.924592</LongitudeDegrees></Position><AltitudeMeters>75.601</AltitudeMeters><DistanceMeters>4429.333</DistanceMeters><Cadence>72</Cadence><Extensions><TPX xmlns=\"http://www.garmin.com/xmlschemas/ActivityExtension/v2\"><Watts>140</Watts></TPX></Extensions></Trackpoint><Trackpoint><Time>2008-03-03T13:56:11Z</Time><Position><LatitudeDegrees>35.875375</LatitudeDegrees><LongitudeDegrees>-78.924499</LongitudeDegrees></Position><AltitudeMeters>76.081</AltitudeMeters><DistanceMeters>4437.728</DistanceMeters><Cadence>77</Cadence><Extensions><TPX xmlns=\"http://www.garmin.com/xmlschemas/ActivityExtension/v2\"><Watts>146</Watts></TPX></Extensions></Trackpoint><Trackpoint><Time>2008-03-03T13:56:12Z</Time><Position><LatitudeDegrees>35.875373</LatitudeDegrees><LongitudeDegrees>-78.924408</LongitudeDegrees></Position><AltitudeMeters>76.081</AltitudeMeters><DistanceMeters>4445.919</DistanceMeters><Cadence>77</Cadence><Extensions><TPX xmlns=\"http://www.garmin.com/xmlschemas/ActivityExtension/v2\"><Watts>144</Watts></TPX></Extensions></Trackpoint><Trackpoint><Time>2008-03-03T13:56:13Z</Time><Position><LatitudeDegrees>35.875371</LatitudeDegrees><LongitudeDegrees>-78.924319</LongitudeDegrees></Position><AltitudeMeters>76.081</AltitudeMeters><DistanceMeters>4453.948</DistanceMeters><Cadence>74</Cadence><Extensions><TPX xmlns=\"http://www.garmin.com/xmlschemas/ActivityExtension/v2\"><Watts>165</Watts></TPX></Extensions></Trackpoint><Trackpoint><Time>2008-03-03T13:56:14Z</Time><Position><LatitudeDegrees>35.875371</LatitudeDegrees><LongitudeDegrees>-78.924232</LongitudeDegrees></Position><AltitudeMeters>76.081</AltitudeMeters><DistanceMeters>4461.861</DistanceMeters><Cadence>73</Cadence><Extensions><TPX xmlns=\"http://www.garmin.com/xmlschemas/ActivityExtension/v2\"><Watts>175</Watts></TPX></Extensions></Trackpoint><Trackpoint><Time>2008-03-03T13:56:15Z</Time><Position><LatitudeDegrees>35.875371</LatitudeDegrees><LongitudeDegrees>-78.924145</LongitudeDegrees></Position><AltitudeMeters>76.081</AltitudeMeters><DistanceMeters>4469.677</DistanceMeters><Cadence>72</Cadence><Extensions><TPX xmlns=\"http://www.garmin.com/xmlschemas/ActivityExtension/v2\"><Watts>207</Watts></TPX></Extensions></Trackpoint><Trackpoint><Time>2008-03-03T13:56:16Z</Time><Position><LatitudeDegrees>35.875371</LatitudeDegrees><LongitudeDegrees>-78.924059</LongitudeDegrees></Position><AltitudeMeters>76.081</AltitudeMeters><DistanceMeters>4477.463</DistanceMeters><Cadence>72</Cadence><Extensions><TPX xmlns=\"http://www.garmin.com/xmlschemas/ActivityExtension/v2\"><Watts>204</Watts></TPX></Extensions></Trackpoint><Trackpoint><Time>2008-03-03T13:56:17Z</Time><Position><LatitudeDegrees>35.875371</LatitudeDegrees><LongitudeDegrees>-78.923972</LongitudeDegrees></Position><AltitudeMeters>76.562</AltitudeMeters><DistanceMeters>4485.291</DistanceMeters><Cadence>73</Cadence><Extensions><TPX xmlns=\"http://www.garmin.com/xmlschemas/ActivityExtension/v2\"><Watts>207</Watts></TPX></Extensions></Trackpoint><Trackpoint><Time>2008-03-03T13:56:18Z</Time><Position><LatitudeDegrees>35.875371</LatitudeDegrees><LongitudeDegrees>-78.923886</LongitudeDegrees></Position><AltitudeMeters>76.562</AltitudeMeters><DistanceMeters>4493.082</DistanceMeters><Cadence>72</Cadence><Extensions><TPX xmlns=\"http://www.garmin.com/xmlschemas/ActivityExtension/v2\"><Watts>204</Watts></TPX></Extensions></Trackpoint><Trackpoint><Time>2008-03-03T13:56:19Z</Time><Position><LatitudeDegrees>35.875373</LatitudeDegrees><LongitudeDegrees>-78.923800</LongitudeDegrees></Position><AltitudeMeters>77.043</AltitudeMeters><DistanceMeters>4500.833</DistanceMeters><Cadence>72</Cadence><Extensions><TPX xmlns=\"http://www.garmin.com/xmlschemas/ActivityExtension/v2\"><Watts>208</Watts></TPX></Extensions></Trackpoint><Trackpoint><Time>2008-03-03T13:56:20Z</Time><Position><LatitudeDegrees>35.875376</LatitudeDegrees><LongitudeDegrees>-78.923715</LongitudeDegrees></Position><AltitudeMeters>77.043</AltitudeMeters><DistanceMeters>4508.562</DistanceMeters><Cadence>71</Cadence><Extensions><TPX xmlns=\"http://www.garmin.com/xmlschemas/ActivityExtension/v2\"><Watts>211</Watts></TPX></Extensions></Trackpoint><Trackpoint><Time>2008-03-03T13:56:21Z</Time><Position><LatitudeDegrees>35.875378</LatitudeDegrees><LongitudeDegrees>-78.923630</LongitudeDegrees></Position><AltitudeMeters>77.043</AltitudeMeters><DistanceMeters>4516.128</DistanceMeters><Cadence>70</Cadence><Extensions><TPX 
